vi "Set_LS3XX.vi"(7 "LS336FrontPanel.vi":bool, 8 "error in (no error)":errorcluster, 11 "Message_command in":T1) -> (0 "error out":errorcluster, 3 "Message_command out":T1)   [LabVIEW 2021]
uses:
  Command_Message.ctl
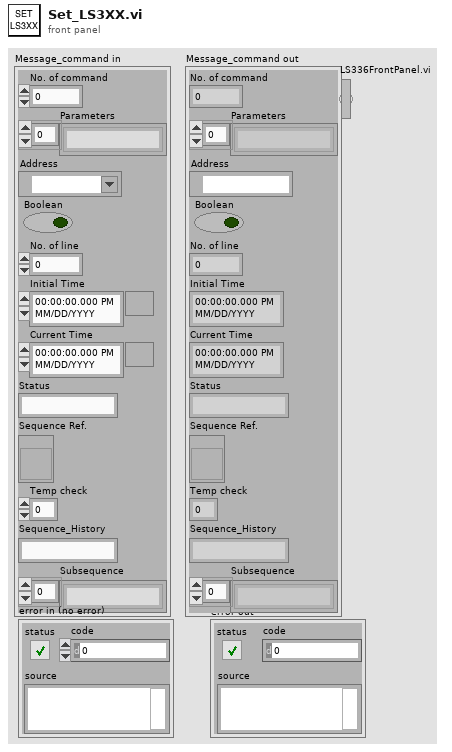
[diagram p1: front panel]
types:
  T1 = typedef "Command_Message.ctl" = cluster{"No. of command":i32, "Parameters":string[], "Address":refnum<visa-resource-name>, "Boolean":bool, "No. of line":i32, "Initial Time":timestamp, "Current Time":timestamp, "Status":string, "Sequence Ref.":refnum<vi>, "Temp check":i32, "Sequence_History":string, "Subsequence":string[]}
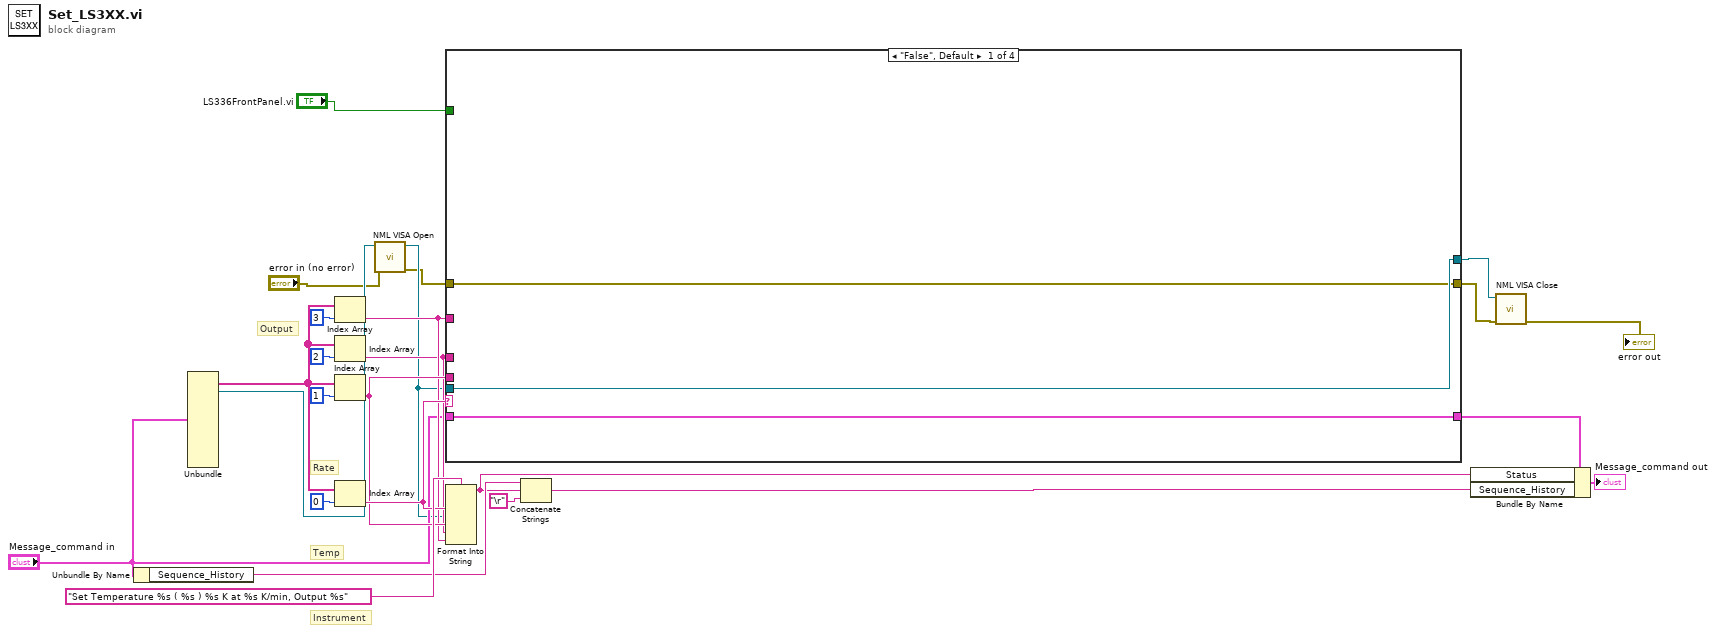
[diagram p0: block diagram]
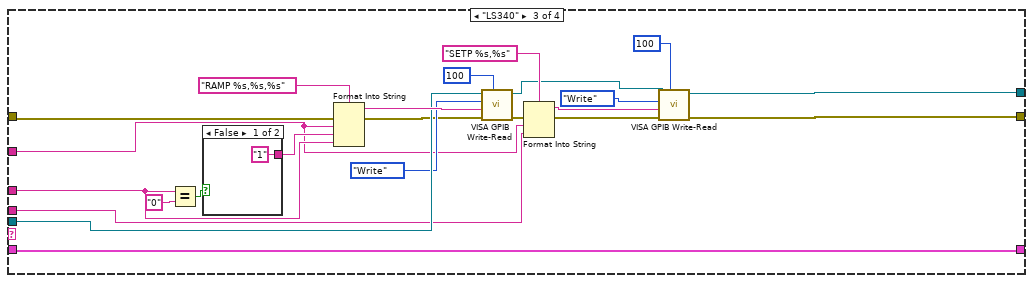
[diagram p3: hidden frame]
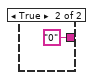
[diagram p4: hidden frame]
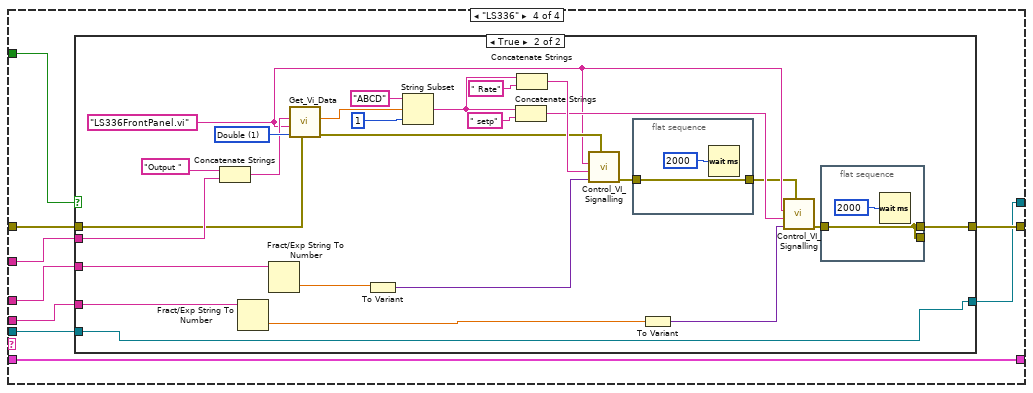
[diagram p5: hidden frame]
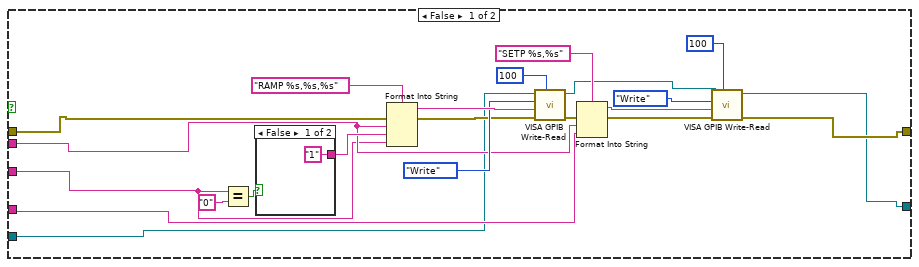
[diagram p6: hidden frame]
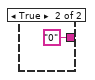
[diagram p7: hidden frame]
diagram:
  # "Instrument"
  # "Temp"
  # "Rate"
  # "Output"
  n1 = Unbundle By Name("Message_command in") -> ("Sequence_History"=w12:string)
  n2 = Unbundle("Message_command in") -> ("Parameters"=w21:string[], "Address"=w7:refnum<visa-resource-name>)  [unwired: 10 out]
  n3 = Index Array(array=w21, index=3) -> (element=w17:string)
  n4 = Index Array(array=w21, index=2) -> (element=w16:string)
  n5 = Index Array(array=w21, index=1) -> (element=w18:string)
  n6 = Index Array(array=w21, index=0) -> (element=w19:string)
  n7 = call "NML VISA Open.vi"("error in (no error)"="error in (no error)", "VISA resource name"=w7) -> ("error out"=w1:errorcluster, "VISA resource name out"=w6:refnum<visa-resource-name>)  [unwired: 8 in]
  n8 = case shown="\"False\", Default" w19 {
    tunnel: w16 -> [_ _ w50 w62]
    tunnel: w17 -> [_ _ w40 w64]
    tunnel: w1 -> [w27 w30 w49 w63]
    tunnel: w6 -> [w28 w31 w47 w58]
    tunnel: w18 -> [_ _ w39 w61]
    tunnel: [w27 w30 w34 w60] -> w4
    tunnel: [w28 w31 w33 w57] -> w5
    tunnel: "Message_command in" -> [w26 w29 w32 w65]
    tunnel: [w26 w29 w32 w65] -> w15
    tunnel: "LS336FrontPanel.vi" -> [_ _ _ w59]
    frame "False", Default {
    }
    frame "LS370" {
    }
    frame "LS340" {
      n9 = Equal?(x=w50, y="0") -> (x = y?=w53:bool)
      n10 = case shown="False" w53 {
        tunnel: ["1" "0"] -> w51
        frame False {
        }
        frame True {
        }
      }
      n11 = Format Into String(format string="RAMP %s,%s,%s", error in=w49, w40, w51, w50) -> (resulting string=w48:string, error out=w42:errorcluster)  [unwired: 1 in]
      n12 = call "VISA GPIB Write-Read.vi"("Wait (ms)"=u32 100 ("wait (mS)"), "error in (no error)"=w42, "Command"=w48, "Action"=enum16{"Write", "Read", "Write & Read"}."Write", "VISA resource name"=w47) -> ("error out"=w41:errorcluster, "dup VISA Session"=w43:refnum<visa-resource-name>)  [unwired: 3 in, 2 out]
      n13 = Format Into String(format string="SETP %s,%s", error in=w41, w40, w39) -> (resulting string=w36:string, error out=w38:errorcluster)  [unwired: 1 in]
      n14 = call "VISA GPIB Write-Read.vi"("Wait (ms)"=u32 100 ("wait (mS)"), "error in (no error)"=w38, "Command"=w36, "Action"=enum16{"Write", "Read", "Write & Read"}."Write", "VISA resource name"=w43) -> ("error out"=w34:errorcluster, "dup VISA Session"=w33:refnum<visa-resource-name>)  [unwired: 3 in, 2 out]
    }
    frame "LS336" {
      n15 = case shown="True" w59 {
        tunnel: w64 -> [w71 w110]
        tunnel: w63 -> [w72 w107]
        tunnel: w62 -> [w70 w102]
        tunnel: w61 -> [w69 w97]
        tunnel: [w67 w91] -> w60
        tunnel: w58 -> [w68 w90]
        tunnel: [w66 w90] -> w57
        frame False {
          n16 = Equal?(x=w70, y="0") -> (x = y?=w86:bool)
          n17 = case shown="False" w86 {
            tunnel: ["1" "0"] -> w84
            frame False {
            }
            frame True {
            }
          }
          n18 = Format Into String(format string="RAMP %s,%s,%s", error in=w72, w71, w84, w70) -> (resulting string=w83:string, error out=w78:errorcluster)  [unwired: 1 in]
          n19 = call "VISA GPIB Write-Read.vi"("Wait (ms)"=u32 100 ("wait (mS)"), "error in (no error)"=w78, "Command"=w83, "Action"=enum16{"Write", "Read", "Write & Read"}."Write", "VISA resource name"=w68) -> ("error out"=w77:errorcluster, "dup VISA Session"=w79:refnum<visa-resource-name>)  [unwired: 3 in, 2 out]
          n20 = Format Into String(format string="SETP %s,%s", error in=w77, w71, w69) -> (resulting string=w74:string, error out=w76:errorcluster)  [unwired: 1 in]
          n21 = call "VISA GPIB Write-Read.vi"("Wait (ms)"=u32 100 ("wait (mS)"), "error in (no error)"=w76, "Command"=w74, "Action"=enum16{"Write", "Read", "Write & Read"}."Write", "VISA resource name"=w79) -> ("error out"=w67:errorcluster, "dup VISA Session"=w66:refnum<visa-resource-name>)  [unwired: 3 in, 2 out]
        }
        frame True {
          w115 = u16 1 items=["String", "Double", "Boolean", "Variant"] ("Data Type")
          w98 = "LS336FrontPanel.vi" ("Target VI name")
          n22 = Concatenate Strings("Output " ("string"), w110) -> (w109:string)
          n23 = Fract/Exp String To Number(string=w97) -> (number=w96:dbl)  [unwired: 3 in, 1 out]
          n24 = Fract/Exp String To Number(string=w102) -> (number=w105:dbl)  [unwired: 3 in, 1 out]
          n25 = call "Get_Vi_Data.vi"("error in (no error) 2"=w107, "Data Type"=w115, "VI name"=w98, "Control Name"=w109) -> ("error out"=w103:errorcluster, "Data (Double)"=w113:dbl)  [unwired: 3 in, 3 out]
          n26 = To Variant(anything=w105) -> (Variant=w104:variant)
          n27 = String Subset(string="ABCD", offset (0)=w113, length (rest)=1 ("length (rest)")) -> (substring=w100:string)
          n28 = Concatenate Strings(w100, " setp" ("string")) -> (w99:string)
          n29 = Concatenate Strings(w100, " Rate" ("string")) -> (w106:string)
          n30 = call "Control_VI_Signalling.vi"("error in (no error)"=w103, "Input Value"=w104, "Control Name"=w106, "Target VI name"=w98) -> ("error out"=w94:errorcluster)  [unwired: 7 in]
          n31 = flat-sequence {
            tunnel: w94 -> [w118]
            tunnel: [w118] -> w93
            frame #0 {
              n32 = Wait (ms)(milliseconds to wait=u32 2000) -> ()  [unwired: 1 out]
            }
          }
          n33 = To Variant(anything=w96) -> (Variant=w95:variant)
          n34 = call "Control_VI_Signalling.vi"("error in (no error)"=w93, "Input Value"=w95, "Control Name"=w99, "Target VI name"=w98) -> ("error out"=w92:errorcluster)  [unwired: 7 in]
          n35 = flat-sequence {
            tunnel: w92 -> [w116]
            tunnel: [w116] -> _
            tunnel: [w116] -> w91
            frame #0 {
              n36 = Wait (ms)(milliseconds to wait=u32 2000) -> ()  [unwired: 1 out]
            }
          }
        }
      }
    }
  }
  n37 = Format Into String(format string="Set Temperature %s ( %s ) %s K at %s K/min, Output %s", w19, w6, w18, w16, w17) -> (resulting string=w11:string)  [unwired: 2 in, 1 out]
  n38 = Concatenate Strings(w12, w11, "\r") -> (w9:string)
  n39 = Bundle By Name(cluster=w15, "Status"=w11, "Sequence_History"=w9) -> (→"Message_command out":T1)
  n40 = call "NML VISA Close.vi"("Error In"=w4, "VISA resource name"=w5) -> ("Error Out"=→"error out":errorcluster)  [unwired: 9 in]
